vi "Allocate.vi"(8 "error in (no error)":errorcluster, 10 "size":u64 format="%d bytes", 11 "Pointer in":refnum<class "Pointer.lvclass">) -> (0 "error out":errorcluster, 3 "Pointer out":refnum<class "Pointer.lvclass">)   [LabVIEW 2017, in "Memory Manager.lvlib" / "Pointer.lvclass"]
uses:
  Pointer.lvclass
  Pointer.lvclass/Pointer.ctl
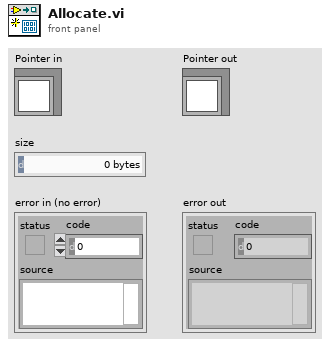
[diagram p1: front panel]
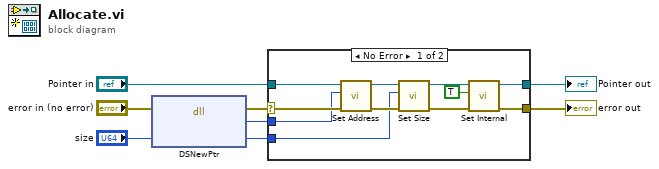
[diagram p0: block diagram]
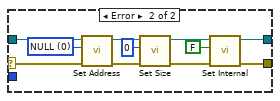
[diagram p2: hidden frame]
diagram:
  n1 = dll-call lib="LabVIEW" fn="DSNewPtr"(error in="error in (no error)", "size"="size") -> (error out=w6:errorcluster, "pointer"=w8:u64, "size"=w7:u64)  [unwired: 2 in, 1 out]
  n2 = case shown="No Error" w6 {
    selector: w6 -> [w16 w21]
    tunnel: "Pointer in" -> [w15 w22]
    tunnel: w8 -> [w14 _]
    tunnel: [w10 w18] -> w5
    tunnel: w7 -> [w12 _]
    tunnel: [w16 w21] -> w3
    frame No Error {
      n3 = call "Set Address.vi"("address"=w14, "Pointer in"=w15) -> ("Pointer out"=w13:refnum<class "Pointer.lvclass">)  [unwired: 9 in]
      n4 = call "Set Size.vi"("size"=w12, "Pointer in"=w13) -> ("Pointer out"=w11:refnum<class "Pointer.lvclass">)  [unwired: 9 in]
      n5 = call "Set Internal.vi"("internal"=TRUE, "Pointer in"=w11) -> ("Pointer out"=w10:refnum<class "Pointer.lvclass">)  [unwired: 9 in]
    }
    frame Error {
      w20 = u64 0 items=["NULL"] ("Null")
      n6 = call "Set Address.vi"("address"=w20, "Pointer in"=w22) -> ("Pointer out"=w23:refnum<class "Pointer.lvclass">)  [unwired: 9 in]
      n7 = call "Set Size.vi"("size"=u64 0, "Pointer in"=w23) -> ("Pointer out"=w19:refnum<class "Pointer.lvclass">)  [unwired: 9 in]
      n8 = call "Set Internal.vi"("internal"=FALSE, "Pointer in"=w19) -> ("Pointer out"=w18:refnum<class "Pointer.lvclass">)  [unwired: 9 in]
    }
  }
  "error out" <- w3
  "Pointer out" <- w5
